vi "Read Capacitive Touch Buttons.vi"(8 "error in (no error)":errorcluster, 11 "ExplorerHatPro in":refnum<class "LINX-ExplorerHatPro.lvclass">) -> (0 "error out":errorcluster, 2 "Explorer Hat Buttons":bool[](array[boolean]), 3 "ExplorerHatPro out":refnum<class "LINX-ExplorerHatPro.lvclass">)   [LabVIEW 2020, in "LINX-ExplorerHatPro.lvclass"]
uses:
  LINX-ExplorerHatPro.lvclass
  CAP1208/CAP1208.lvclass
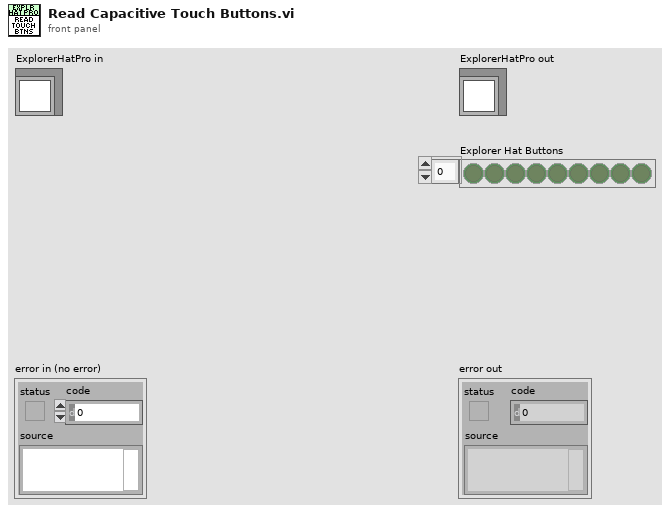
[diagram p1: front panel]
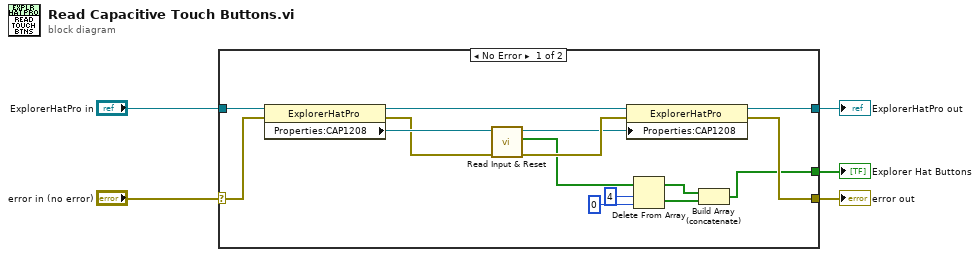
[diagram p0: block diagram]
diagram:
  n1 = case shown="No Error" "error in (no error)" {
    selector: "error in (no error)" -> [w13 w22]
    tunnel: [w12 w22] -> w4
    tunnel: [w18 w21] -> w2
    tunnel: "ExplorerHatPro in" -> [w20 w21]
    tunnel: [w6 _] -> w1
    frame No Error {
      n2 = property class="ExplorerHatPro"(reference=w20, error in=w13) -> (reference out=w19:refnum<class "LINX-ExplorerHatPro.lvclass">, error out=w16:errorcluster, "Properties:CAP1208"=w17:refnum<class "CAP1208.lvclass">)
      n3 = call "Read Input & Reset.vi"("error in (no error)"=w16, "CAP1208 in"=w17) -> ("error out"=w15:errorcluster, "Sensor Input (CS1-CS8)"=w11:bool[], "CAP1208 out"=w14:refnum<class "CAP1208.lvclass">)  [unwired: 6 in, 1 out]
      n4 = property class="ExplorerHatPro"(reference=w19, error in=w15, "Properties:CAP1208"=w14) -> (reference out=w18:refnum<class "LINX-ExplorerHatPro.lvclass">, error out=w12:errorcluster)
      n5 = Delete From Array(array=w11, length=4, index=0) -> (deleted portion=w7:bool[], array with subset deleted=w8:bool[])
      n6 = Build Array (concatenate)(w8, w7) -> (w6:bool[])
    }
    frame Error {
    }
  }
  "error out" <- w4
  "ExplorerHatPro out" <- w2
  "Explorer Hat Buttons" <- w1
